vi "vi.Array2Cluster.vi"(0 "Array":variant[](array[variant]), 11 "error in (no error)":errorcluster) -> (4 "Cluster":variant, 15 "error out":errorcluster)   [LabVIEW 2014, in "GLue.lvlib" / "class.GLue.lvclass"]
uses:
  class.GLue.lvclass
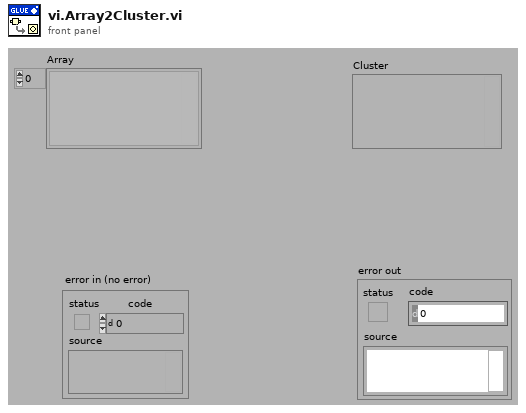
[diagram p1: front panel]
types:
  T1 = enum8{"<Null>", "I8", "I16", "I32", "I64", "U8", "U16", "U32", "U64", "SGL", "DBL", "EXT", "CSG", "CDB", "CXT", "0x0F", "0x10", "0x11", "0x12", "0x13", "0x14", "Enum U8", "Enum U16", "Enum U32", "Enum U64", "SGL PQ", "DBL PQ", "EXT PQ", "CSG PQ", "CDB PQ", "CXT PQ", "0x1F", "0x20", "Boolean", "0x22", "0x23", "0x24", "0x25", "0x26", "0x27", "0x28", "0x29", "0x2A", "0x2B", "0x2C", "0x2D", "0x2E", "0x2F", "String", "0x31", "Path", "Pict", "0x34", "0x35", "0x36", "DAQ", "0x38", "0x39", "0x3A", "0x3B", "0x3C", "0x3D", "0x3E", "0x3F", "Array", "0x41", "0x42", "0x43", "0x44", "0x45", "0x46", "0x47", "0x48", "0x49", "0x4A", "0x4B", "0x4C", "0x4D", "0x4E", "0x4F", "Cluster", "0x51", "0x52", "Variant", "Waveform", "0x55", "0x56", "0x57", "0x58", "0x59", "0x5A", "0x5B", "0x5C", "0x5D", "0x5E", "0x5F", "0x60", "0x61", "0x62", "0x63", "0x64", "0x65", "0x66", "0x67", "0x68", "0x69", "0x6A", "0x6B", "0x6C", "0x6D", "0x6E", "0x6F", "Refnum"}
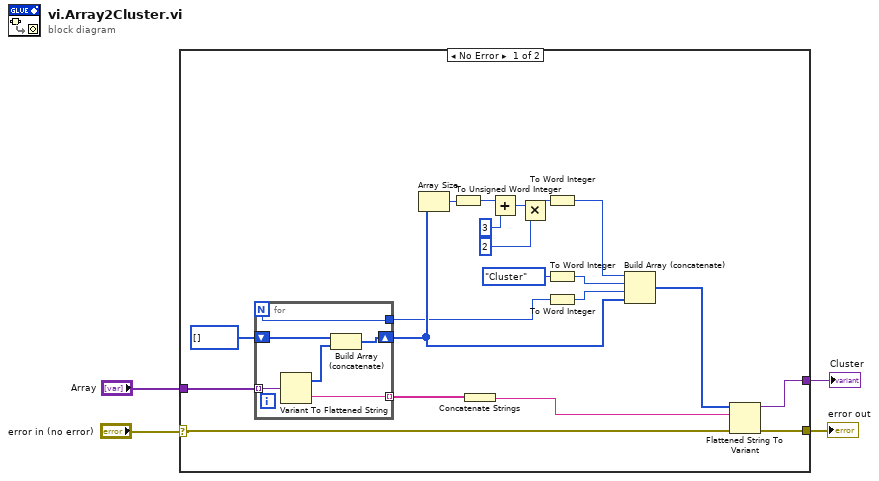
[diagram p0: block diagram]
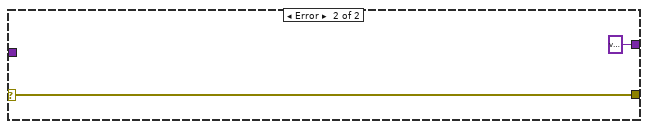
[diagram p2: hidden frame]
diagram:
  n1 = case shown="No Error" "error in (no error)" {
    selector: "error in (no error)" -> [w9 w31]
    tunnel: "Array" -> [w23 _]
    tunnel: [w6 variant ("Variant")] -> w1
    tunnel: [w5 w31] -> w2
    frame No Error {
      n2 = for {
        N -> [w26]
        shift-right: [w27] -> w12
        shift-left: i16[] [] -> [w29]
        tunnel: w23 -> [w30] mode=indexing
        tunnel: [w26] -> w11
        tunnel: [w25] -> w10 mode=indexing
        n3 = Variant To Flattened String(Variant=w30) -> (data string=w25:string, 1:w28:i16[])
        n4 = Build Array (concatenate)(w29, w28) -> (w27:i16[])
      }
      n5 = Array Size(array=w12) -> (size(s)=w13:i32)
      n6 = To Unsigned Word Integer(number=w13) -> (unsigned 16bit integer=w21:u16)
      n7 = Concatenate Strings(w10) -> (w7:string)
      n8 = Add(x=w21, y=u16 3 ("cluster TD header I16s to add")) -> (x+y=w19:u16)
      n9 = Multiply(x=w19, y=u16 2 ("bytes per I16")) -> (x*y=w22:u16)
      n10 = To Word Integer(number=w22) -> (16bit integer=w14:i16)
      n11 = To Word Integer(number=T1."Cluster" ("type")) -> (16bit integer=w17:i16)
      n12 = To Word Integer(number=w11) -> (16bit integer=w16:i16)
      n13 = Build Array (concatenate)(w14, w17, w16, w12) -> (w8:i16[])
      n14 = Flattened String To Variant(4:w9, 6:w7, 7:w8) -> (0:w5:errorcluster, 3:w6:variant)
    }
    frame Error {
    }
  }
  "error out" <- w2
  "Cluster" <- w1
